vi "Element Init.vi"(7 "VolatusAPI":refnum<class "VolatusAPI.lvclass">, 8 "error in (no error)":errorcluster, 10 "JSON":string, 11 "SystemConfigStatusIndicator in":refnum<class "SystemConfigStatusIndicator.lvclass">) -> (0 "error out":errorcluster, 3 "SystemConfigStatusIndicator out":refnum<class "SystemConfigStatusIndicator.lvclass">)   [LabVIEW 2020, in "VolatusGUIElements.lvlib" / "SystemConfigStatusIndicator.lvclass"]
uses:
  SystemConfigStatusIndicator.lvclass
  Volatus/VolatusAPI/VolatusAPI.lvclass
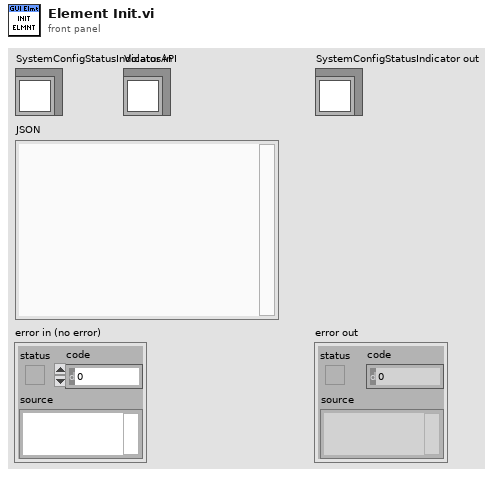
[diagram p1: front panel]
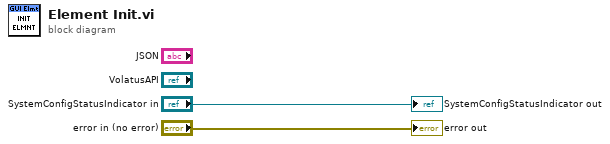
[diagram p0: block diagram]
diagram:
  "error out" <- "error in (no error)"
  "SystemConfigStatusIndicator out" <- "SystemConfigStatusIndicator in"
